vi "Poll Shared Variable.vi"(6 "Reset?":bool, 7 "Message":string, 8 "error in (no error)":errorcluster, 10 "Message handler":refnum<queue>, 11 "Refnum in":refnum<k21>) -> (0 "error out":errorcluster)   [LabVIEW 2014]
uses:
  Message Queue/Message Cluster.ctl
  Message Queue/Message Queue.lvlib
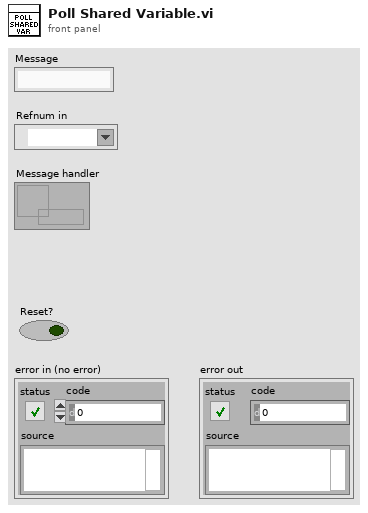
[diagram p1: front panel]
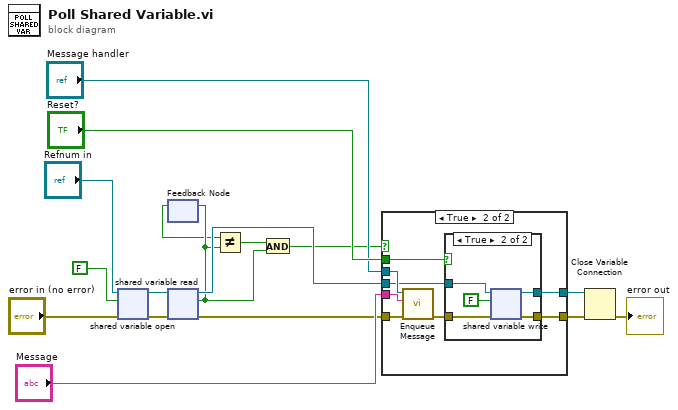
[diagram p0: block diagram]
diagram:
  n1 = shared-variable-open("Refnum in", "error in (no error)", FALSE ("data type")) -> (w3:refnum<k21>, w4:errorcluster)  [unwired: 1 in]
  n2 = feedback #1() -> (w6:bool)  [unwired: 1 in]
  n3 = shared-variable-read(w3, w4) -> (w13:refnum<k21>, w9:errorcluster, w8:bool)  [unwired: 1 out]
  n4 = feedback-in #1(w8) -> ()
  n5 = Not Equal?(x=w6, y=w8) -> (x != y?=w7:bool)
  n6 = And(x=w7, y=w8) -> (x .and. y?=w5:bool)
  n7 = case shown="True" w5 {
    tunnel: [w19 w23] -> w14
    tunnel: w9 -> [w19 w27]
    tunnel: "Message handler" -> [_ w26]
    tunnel: "Message" -> [_ w25]
    tunnel: "Reset?" -> [_ w22]
    tunnel: w13 -> [w18 w21]
    tunnel: [w18 w20] -> w15
    frame False {
    }
    frame True {
      n8 = call "Enqueue Message.vi"("error in (no error)"=w27, "Message"=w25, "Message Queue"=w26) -> ("error out"=w24:errorcluster)  [unwired: 7 in, 1 out]
      n9 = case shown="True" w22 {
        tunnel: w24 -> [w28 w34]
        tunnel: [w28 w33] -> w23
        tunnel: w21 -> [w29 w32]
        tunnel: [w29 w31] -> w20
        frame False {
        }
        frame True {
          n10 = shared-variable-write(w32, w34, FALSE ("data in")) -> (w31:refnum<k21>, w33:errorcluster)
        }
      }
    }
  }
  n11 = Close Variable Connection(8:w14, 11:w15) -> (0:→"error out":errorcluster)
